vi "Temperature Conversion.vi"() -> ()   [LabVIEW 2014]
panel:
  in  "stop":bool
  out "Converted Temperature":dbl
  in  "Initial Temperature":dbl
  in  "Type of Conversion":T1(ring)
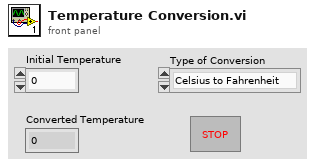
[diagram p1: front panel]
types:
  T1 = enum16{"Celsius to Fahrenheit", "Fahrenheit to Celsius", "Celsius to Kelvin", "Fahrenheit to Kelvin"}
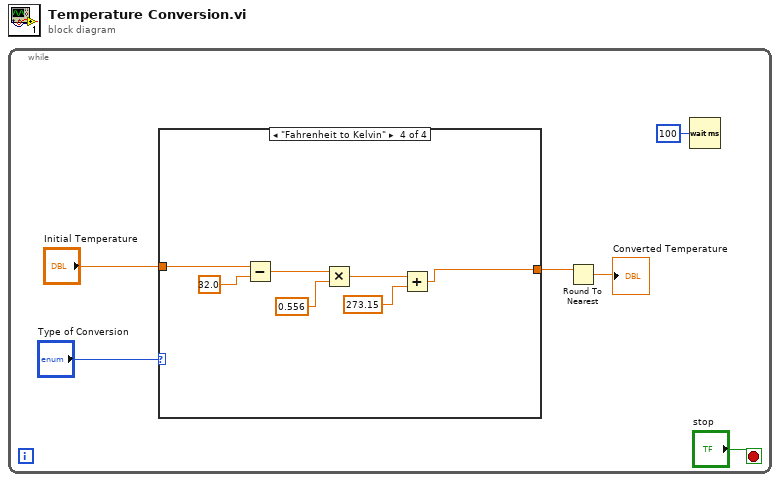
[diagram p0: block diagram]
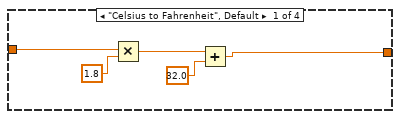
[diagram p2: hidden frame]
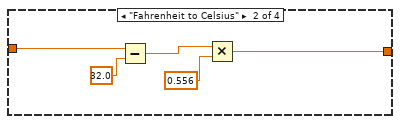
[diagram p3: hidden frame]
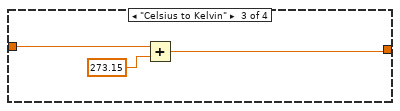
[diagram p4: hidden frame]
diagram:
  n1 = while {
    stop <- "stop" stop-if-true
    n2 = case shown="\"Fahrenheit to Kelvin\"" "Type of Conversion" {
      tunnel: "Initial Temperature" -> [w10 w15 w18 w23]
      tunnel: [w7 w12 w17 w20] -> w4
      frame "Celsius to Fahrenheit", Default {
        n3 = Multiply(x=w10, y=1.8) -> (x*y=w8:dbl)
        n4 = Add(x=w8, y=32.0) -> (x+y=w7:dbl)
      }
      frame "Fahrenheit to Celsius" {
        n5 = Subtract(x=w15, y=32.0) -> (x-y=w13:dbl)
        n6 = Multiply(x=w13, y=0.556) -> (x*y=w12:dbl)
      }
      frame "Celsius to Kelvin" {
        n7 = Add(x=w18, y=273.15) -> (x+y=w17:dbl)
      }
      frame "Fahrenheit to Kelvin" {
        n8 = Subtract(x=w23, y=32.0) -> (x-y=w22:dbl)
        n9 = Multiply(x=w22, y=0.556) -> (x*y=w21:dbl)
        n10 = Add(x=w21, y=273.15) -> (x+y=w20:dbl)
      }
    }
    n11 = Round To Nearest(number=w4) -> (nearest integer value=→"Converted Temperature":dbl)
    n12 = Wait (ms)(milliseconds to wait=u32 100) -> ()  [unwired: 1 out]
  }
